vi "_ADC_ Signal Saturation.vi"(8 "Supply Parameters":T1={"ADC Supply Ripple Frequency"=10.0, "Gen Wave Sampling Frequency"=0.0, "ADC Neg Supply Ripple Amplitude"=0.0, "ADC Neg Supply Offset"=0.0, "ADC Pos Supply Ripple Amplitude"=0.0, "ADC Pos Supply Offset"=0.0, "ADC Supply Diff Noise Amplitude"=0.0}, 11 "Input Wave":waveform(dbl)) -> (3 "Output Wave":waveform(dbl))   [LabVIEW 2014]
uses:
  Ctls/_ADC_ Supply Variables.ctl
  <vilib>/measure/NI_MABase.lvlib
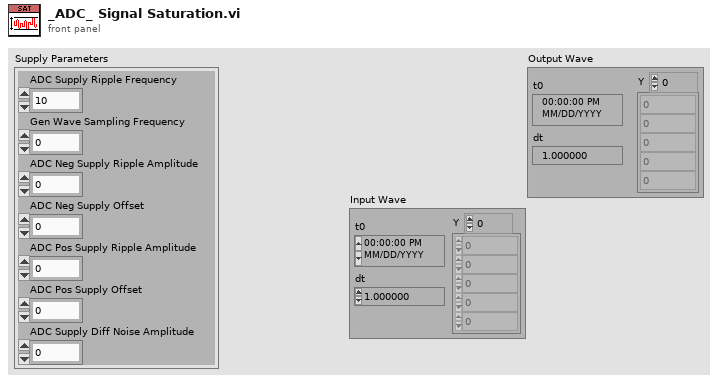
[diagram p1: front panel]
types:
  T1 = typedef "_ADC_ Supply Variables.ctl" = cluster{"ADC Supply Ripple Frequency":dbl, "Gen Wave Sampling Frequency":dbl, "ADC Neg Supply Ripple Amplitude":dbl, "ADC Neg Supply Offset":dbl, "ADC Pos Supply Ripple Amplitude":dbl, "ADC Pos Supply Offset":dbl, "ADC Supply Diff Noise Amplitude":dbl}
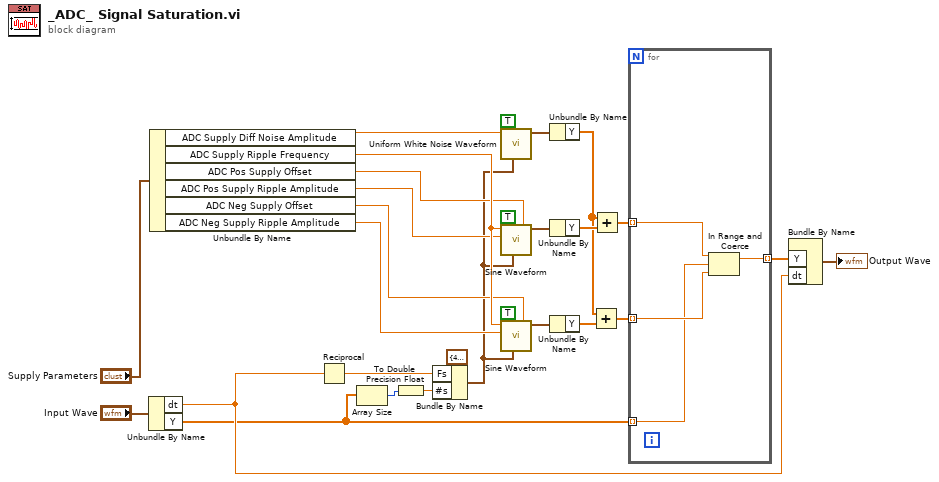
[diagram p0: block diagram]
diagram:
  n1 = Unbundle By Name("Input Wave") -> ("dt"=w7:dbl, "Y"=w4:dbl[])
  n2 = Unbundle By Name("Supply Parameters") -> ("ADC Supply Diff Noise Amplitude"=w22:dbl, "ADC Supply Ripple Frequency"=w21:dbl, "ADC Pos Supply Offset"=w20:dbl, "ADC Pos Supply Ripple Amplitude"=w19:dbl, "ADC Neg Supply Offset"=w18:dbl, "ADC Neg Supply Ripple Amplitude"=w17:dbl)
  n3 = Reciprocal(x=w7) -> (1/x=w8:dbl)
  n4 = Array Size(array=w4) -> (size(s)=w3:i32)
  n5 = To Double Precision Float(number=w3) -> (double precision float=w2:dbl)
  n6 = Bundle By Name(cluster=cluster{"Fs":dbl, "#s":dbl} {"Fs"=44100.0, "#s"=4410.0} ("Spl Info"), "Fs"=w8, "#s"=w2) -> (w16:cluster{"Fs":dbl, "#s":dbl})
  n7 = call <vilib>:"Uniform White Noise Waveform.vi"("sampling info"=w16, "reset signal"=TRUE, "amplitude"=w22) -> ("signal out"=w26:waveform(dbl))  [unwired: 7 in, 1 out]
  n8 = call <vilib>:"Sine Waveform.vi"("offset"=w20, "sampling info"=w16, "reset signal"=TRUE, "amplitude"=w19, "frequency"=w21) -> ("signal out"=w27:waveform(dbl))  [unwired: 5 in, 1 out]
  n9 = call <vilib>:"Sine Waveform.vi"("offset"=w18, "sampling info"=w16, "reset signal"=TRUE, "amplitude"=w17, "frequency"=w21) -> ("signal out"=w28:waveform(dbl))  [unwired: 5 in, 1 out]
  n10 = Unbundle By Name(w26) -> ("Y"=w13:dbl[])
  n11 = Unbundle By Name(w27) -> ("Y"=w14:dbl[])
  n12 = Unbundle By Name(w28) -> ("Y"=w15:dbl[])
  n13 = Add(x=w13, y=w15) -> (x+y=w11:dbl[])
  n14 = Add(x=w13, y=w14) -> (x+y=w12:dbl[])
  n15 = for {
    tunnel: w12 -> [w32] mode=indexing
    tunnel: w11 -> [w31] mode=indexing
    tunnel: [w30] -> w6 mode=indexing
    tunnel: w4 -> [w29] mode=indexing
    n16 = In Range and Coerce(upper limit=w32, x=w29, lower limit=w31) -> (coerced(x)=w30:dbl)  [unwired: 1 out]
  }
  n17 = Bundle By Name("Y"=w6, "dt"=w7) -> (→"Output Wave":waveform(dbl))  [unwired: 1 in]
